vi "AddNewNode.vi"(4 "Cancel":bool, 6 "Attributes":string[][](array[string]), 8 "Insert As Child":bool, 9 "New Node Name":string, 10 "Node ID":string, 11 "DOM document":refnum<k20>) -> ()   [LabVIEW 2017]
uses:
  <vilib>/xml/NI_XML.lvlib
  <resource>/objmgr/DOMUserDefRef.rc
panel:
  out "appended array":string[][](array[string])
  out "XML":string
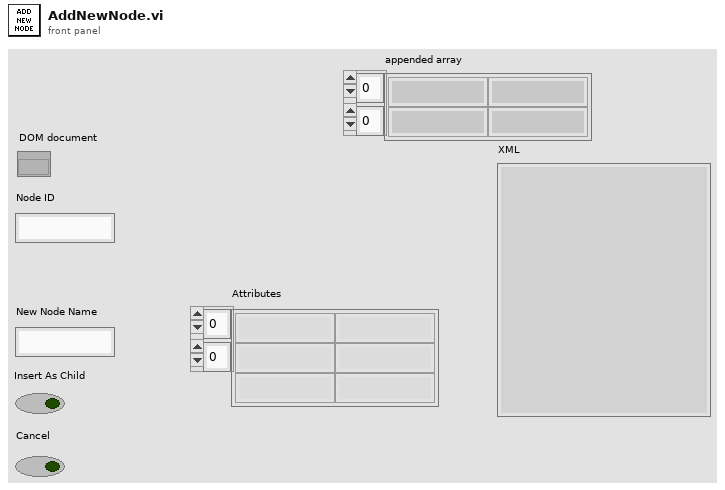
[diagram p1: front panel]
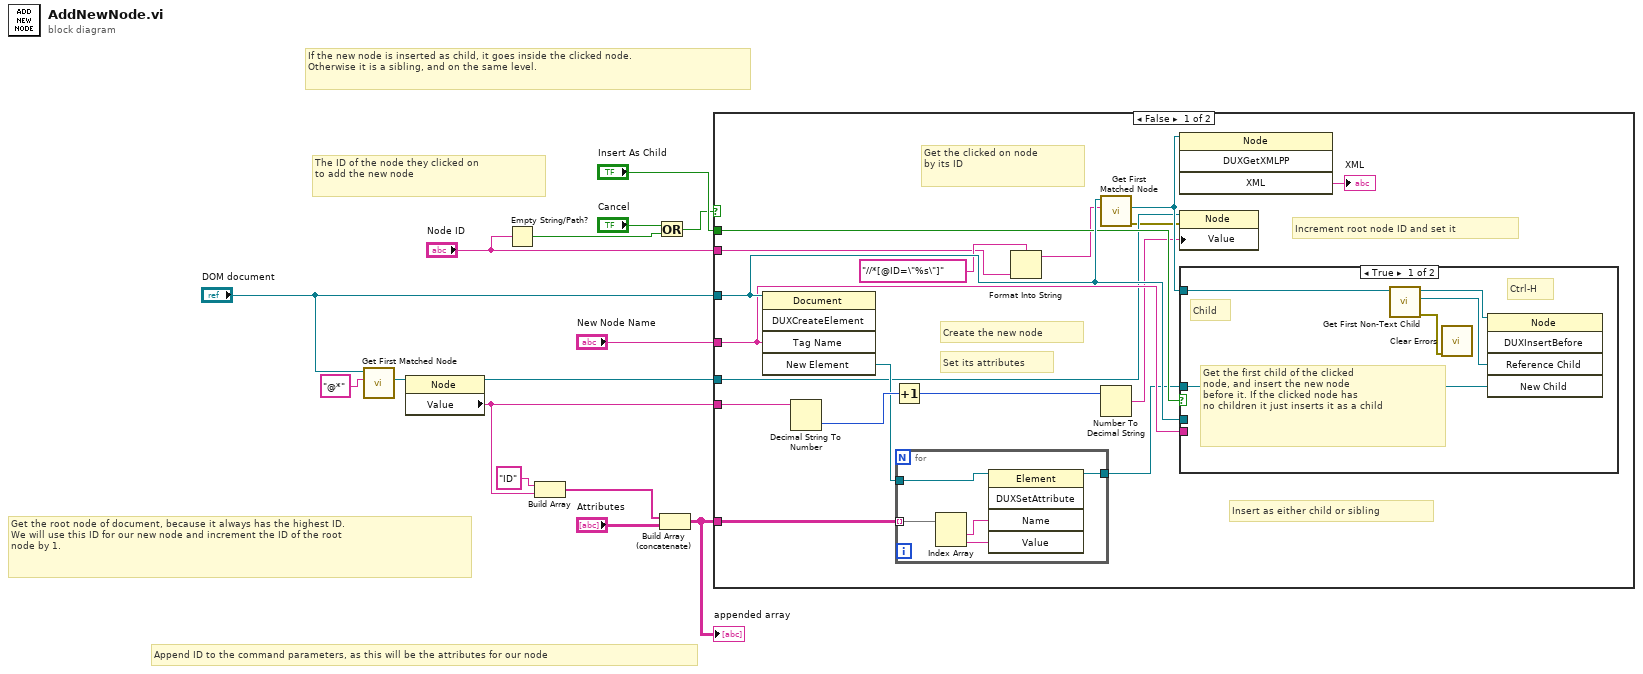
[diagram p0: block diagram]
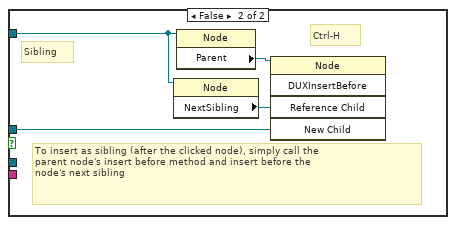
[diagram p2: hidden frame]
diagram:
  # "The ID of the node they clicked on\nto add the new node"
  # "If the new node is inserted as child, it goes inside the clicked node.\nOtherwise it is a sibling, and on the same level."
  # "Append ID to the command parameters, as this will be the attributes for our node"
  # "Get the root node of document, because it always has the highest ID.\nWe will use this ID for our new node and increment the ID of the root\nnode by 1."
  n1 = call <vilib>:"Get First Matched Node.vi"("XPath expression"="@*", "node in"="DOM document") -> ("node result"=w10:refnum<k20>)  [unwired: 7 in, 2 out]
  n2 = property class="Node"(reference=w10) -> (reference out=w8:refnum<k20>, "Value"=w5:string)  [unwired: 1 in, 1 out]
  n3 = Empty String/Path?(string/path="Node ID") -> (empty?=w3:bool)
  n4 = Build Array("ID" ("XPath expression"), w5) -> (w11:string[])
  n5 = Or(x="Cancel", y=w3) -> (x .or. y?=w1:bool)
  n6 = Build Array (concatenate)(w11, "Attributes") -> (w4:string[][])
  "appended array" <- w4
  n7 = case shown="False" w1 {
    tunnel: "DOM document" -> [w32 _]
    tunnel: "Insert As Child" -> [w31 _]
    tunnel: "New Node Name" -> [w30 _]
    tunnel: "Node ID" -> [w22 _]
    tunnel: w8 -> [w19 _]
    tunnel: w5 -> [w18 _]
    tunnel: w4 -> [w17 _]
    frame False {
      # "Insert as either child or sibling"
      # "Get the clicked on node\nby its ID"
      # "Increment root node ID and set it"
      # "Set its attributes"
      # "Create the new node"
      n8 = invoke class="Document" method="DUXCreateElement"(reference=w32, "Tag Name"=w30) -> ("New Element"=w21:refnum<k20>)  [unwired: 3 in, 4 out]
      n9 = Decimal String To Number(string=w18) -> (number=w23:i32)  [unwired: 2 in, 1 out]
      n10 = Increment(x=w23) -> (x+1=w24:i32)
      n11 = for {
        tunnel: w21 -> [w37]
        tunnel: [w36] -> w20
        tunnel: w17 -> [w35] mode=indexing
        n12 = Index Array(array=w35) -> (element #1=w34:string, element #2=w33:string)  [unwired: 2 in]
        n13 = invoke class="Element" method="DUXSetAttribute"(reference=w37, "Name"=w34, "Value"=w33) -> (reference out=w36:refnum<k20>)  [unwired: 2 in, 4 out]
      }
      n14 = Format Into String(format string="//*[@ID=\"%s\"]", w22) -> (resulting string=w26:string)  [unwired: 2 in, 1 out]
      n15 = call <vilib>:"Get First Matched Node.vi"("XPath expression"=w26, "node in"=w32) -> ("error out"=w16:errorcluster, "node result"=w28:refnum<k20>)  [unwired: 7 in, 1 out]
      n16 = Number To Decimal String(number=w24) -> (decimal integer string=w25:string)  [unwired: 1 in]
      n17 = invoke class="Node" method="DUXGetXMLPP"(reference=w28) -> ("XML"=→"XML":string)  [unwired: 3 in, 3 out]
      n18 = property class="Node"(reference=w19, error in=w16, "Value"=w25) -> ()  [unwired: 2 out]
      n19 = case shown="True" w31 {
        tunnel: w32 -> [_ _]
        tunnel: w30 -> [_ _]
        tunnel: w28 -> [w39 w45]
        tunnel: w20 -> [w38 w43]
        frame True {
          # "Ctrl-H"
          # "Get the first child of the clicked\nnode, and insert the new node \nbefore it. If the clicked node has\nno children it just inserts it as a child"
          # "Child"
          n20 = call <vilib>:"Get First Non-Text Child.vi"("node in"=w39) -> ("error out"=w40:errorcluster, "child node"=w41:refnum<k20>, "node out"=w42:refnum<k20>)  [unwired: 7 in, 1 out]
          n21 = call <vilib>:"Clear Errors.vi"("error in (no error)"=w40) -> ()  [unwired: 5 in, 2 out]
          n22 = invoke class="Node" method="DUXInsertBefore"(reference=w42, "Reference Child"=w41, "New Child"=w38) -> ()  [unwired: 2 in, 5 out]
        }
        frame False {
          # "Ctrl-H"
          # "To insert as sibling (after the clicked node), simply call the\nparent node's insert before method and insert before the \nnode's next sibling"
          # "Sibling"
          n23 = property class="Node"(reference=w45) -> ("NextSibling"=w46:refnum<k20>)  [unwired: 1 in, 2 out]
          n24 = property class="Node"(reference=w45) -> ("Parent"=w44:refnum<k20>)  [unwired: 1 in, 2 out]
          n25 = invoke class="Node" method="DUXInsertBefore"(reference=w44, "Reference Child"=w46, "New Child"=w43) -> ()  [unwired: 2 in, 5 out]
        }
      }
    }
    frame True {
      # "If the node they clicked on's ID is empty (not a valid node)\nor the cancel button was pressed when entering\nattributes, don't add the node"
    }
  }
